vi "SP_FORLOOP.vi"(3 "Commands":string[](array[string])) -> (1 "Commands Out":string[](array[string]))   [LabVIEW 2009]
panel:
  # "This LabVIEW item is deprecated.\n\nIt is believed to be unused and will be removed in a future version of SRV."
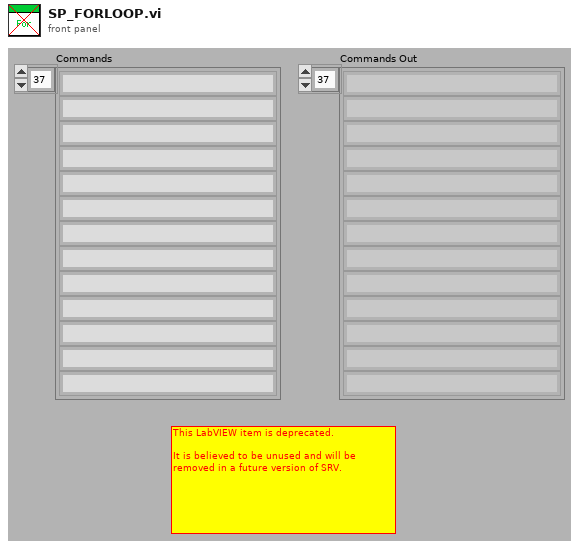
[diagram p1: front panel]
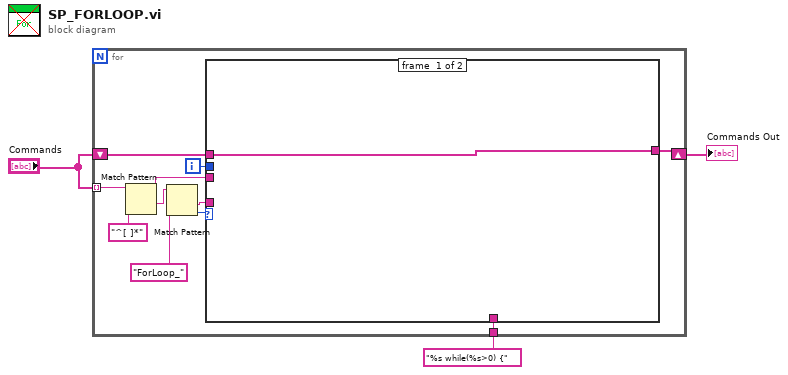
[diagram p0: block diagram]
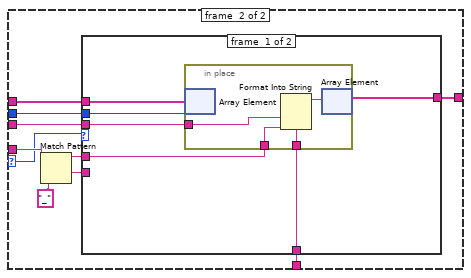
[diagram p2: hidden frame]
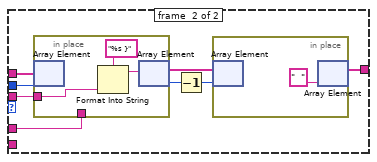
[diagram p3: hidden frame]
diagram:
  n1 = for {
    tunnel: "Commands" -> [w9] mode=indexing
    shift-right: [w10] -> w2
    shift-left: "Commands" -> [w12]
    tunnel: "%s while(%s>0) {" ("format string") -> [w4]
    i -> [w11]
    n2 = Match Pattern(string=w9, regular expression="^[ ]*") -> (match substring=w6:string, after substring=w8:string)  [unwired: 1 in, 2 out]
    n3 = Match Pattern(string=w8, regular expression="ForLoop_") -> (after substring=w13:string, offset past match=w5:i32)  [unwired: 1 in, 2 out]
    n4 = case shown="Default" w5 {
      selector: w5 -> [_ w17]
      tunnel: w13 -> [_ w22]
      tunnel: w12 -> [w15 w25]
      tunnel: w11 -> [_ w24]
      tunnel: [w15 w23] -> w10
      tunnel: w6 -> [_ w18]
      tunnel: w4 -> [_ w16]
      frame #0 {
      }
      frame #1 {
        n5 = Match Pattern(string=w22, regular expression="_") -> (before substring=w20:string, after substring=w19:string)  [unwired: 1 in, 2 out]
        n6 = case shown="Default" w17 {
          tunnel: w25 -> [w31 w43]
          tunnel: w24 -> [w30 w42]
          tunnel: [w29 w38] -> w23
          tunnel: w20 -> [w28 w41]
          tunnel: w19 -> [_ _]
          tunnel: w18 -> [w27 w40]
          tunnel: w16 -> [w26 _]
          frame #0 {
            n7 = in-place {
              in-place-border: w28 -> [w33]
              in-place-border: w27 -> [w35]
              in-place-border: w26 -> [w32]
              n8 = in-place-array #1(w31, w30) -> ()  [unwired: 1 out]
              n9 = Format Into String(format string=w32, w35, w33) -> (resulting string=w34:string)  [unwired: 2 in, 1 out]
              n10 = in-place-array #1(w34) -> (w29:string[])  [unwired: 1 out]
            }
          }
          frame #1 {
            n11 = in-place {
              in-place-border: w41 -> [_]
              in-place-border: w40 -> [w47]
              n12 = in-place-array #2(w43, w42) -> ()  [unwired: 1 out]
              n13 = Format Into String(format string="%s }", w47) -> (resulting string=w46:string)  [unwired: 2 in, 1 out]
              n14 = in-place-array #2(w46) -> (w39:string[], w37:i32)
            }
            n15 = Decrement(x=w37) -> (x-1=w36:i32)
            n16 = in-place {
              n17 = in-place-array #3(w39, w36) -> ()  [unwired: 1 out]
              n18 = in-place-array #3("  " ("format string")) -> (w38:string[])  [unwired: 1 out]
            }
          }
        }
      }
    }
  }
  "Commands Out" <- w2
